vi "Log Model State.vi"(8 "error in (no error)":errorcluster, 10 "Message Data":variant, 11 "Message Queue":refnum<queue>) -> (0 "error out":errorcluster)   [LabVIEW 2015, in "Logger.lvlib"]
uses:
  Logger.lvlib
  support/Message Queue/Message Cluster.ctl
  support/Message Queue/Message Queue.lvlib
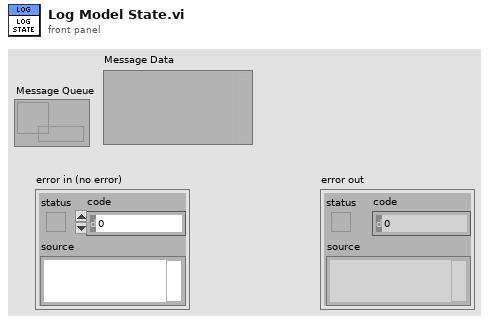
[diagram p1: front panel]
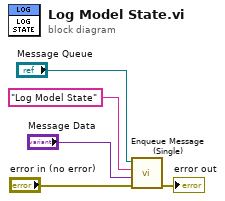
[diagram p0: block diagram]
diagram:
  n1 = call "Enqueue Message (Single).vi"("error in (no error)"="error in (no error)", "Message Data"="Message Data", "Message"="Log Model State", "Message Queue"="Message Queue") -> ("error out"=→"error out":errorcluster)  [unwired: 6 in, 1 out]
